vi "Append LF.vi"(0 "PDF Report IN":T21(xcontrol), 1 "Number of LF (default 1)":u8=1, 11 "error in (no error)":errorcluster) -> (4 "PDF Report duplicate":T21(xcontrol), 15 "error out":errorcluster)   [LabVIEW 2012]
doc: "Appends <B>Line Feed</B> to the PDF report.\n\n<B>FRANÇAIS</B>\nAjoute des <B>sauts de ligne</B> au rapport PDF.\n\nDeveloped by Jean-Marc Simard\nCopyright © 2010, Exaprom Inc.\nAll rights reserved.\nLicense: BSD\n\nWith iTextSharp 4.1.6 (http://itextsharp.sourceforge.net)\nunder Mozilla Public License Version 1.1\n(http://www.mozilla.org/MPL/MPL-1.1.html)"
uses:
  Controls/PDF Report Xcontrol/PDF Report.xctl
  C:/Users/MaxCorp/Documents/TopPerm - Base/DLL/itextsharp.dll
  DLL/itextsharp.dll
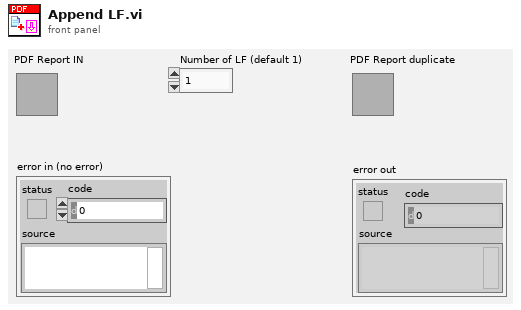
[diagram p1: front panel]
types:
  T1 = typedef "Font cluster.ctl" = cluster{"Name":string, "Size":T2, "Color":T3, "Style":cluster{"Bold":bool, "Italic":bool, "Underline":bool, "Strikeout":bool}}
  T2 = typedef "Font size.ctl" = sgl
  T3 = typedef "Font color.ctl" = u32
  T4 = typedef "Unit.ctl" = enum16{"inch", "mm"}
  T5 = typedef "Paragraphe cluster.ctl" = cluster{" Aligment":T6, "Line spacing":T7}
  T6 = typedef "Texte alignement.ctl" = enum16{"Select", "CENTER", "JUSTIFY", "LEFT", "RIGHT"}
  T7 = typedef "Line spacing.ctl" = enum16{"Select", "1.0", "1.5", "2.0"}
  T8 = typedef "Page dimensions.ctl" = cluster{"Start at page":i32, "Orientation":T9, "widht":sgl, "height":sgl, "Margin left":sgl, "Margin right":sgl, "Margin top":sgl, "Margin bottom":sgl}
  T9 = typedef "Page Orientation.ctl" = enum16{"Portrait", "Landscape"}
  T10 = typedef "Image or Table Caption.ctl" = cluster{"Caption":string, "Separator":string, "Position":enum16{"Above", "Below"}}
  T11 = typedef "Header Footer [ ].ctl" = T12[]
  T12 = typedef "Header Footer cluster.ctl" = cluster{"Start page":i32, "Type":T13, "Alignment":T14, "Vertical Alignement":T15, "Image (%)":sgl, "Page #":T16, "Text":string, "Path":string, "Font":T1, "Font refnum":refnum<k24>, "Line":cluster{"Line":T17, "Thickness (points)":sgl, "Colour":T3}}
  T13 = typedef "Header Footer Type.ctl" = enum16{"Select", "Text", "Text + hyperlink", "Page number", "Image", "Image + hyperlink"}
  T14 = typedef "Header footer horiz alignment.ctl" = enum16{"Left", "Center", "Right"}
  T15 = typedef "Cell Vertical alignment.ctl" = enum16{"TOP", "MIDDLE", "BOTTOM"}
  T16 = typedef "Page number.ctl" = cluster{"Text 1":string, "Text 2":string, "Text 3":string}
  T17 = typedef "Header Footer Line.ctl" = enum16{"No line", "Horizontal line"}
  T18 = typedef "Watermark cluster2.ctl" = cluster{"Show? (F)":bool, "Type":enum16{"Image", "Text"}, "Opacity (%)":sgl, "Rotate(°)":sgl, "Position":cluster{"Position":T19, "X":sgl, "Y":sgl}, "Image path":path, "Scaled(%)":sgl, "Image refnum":refnum<k24>, "Text":string, "Font":cluster{"Name":string, "Size":T2, "Color":T3}, "Font refnum":refnum<k24>, "Alignment":T14, "Automatic":bool}
  T19 = typedef "Watermark Position.ctl" = enum16{"Absolute", "Center (page)", "Center (text section)"}
  T20 = typedef "System Fonts.ctl" = cluster{"Font name [ ]":string[], "Font and file names [ ]":cluster{"Font name":string, "File name":string}[]}
  T21 = cluster{"Document":refnum<k24>, "Writer":refnum<k24>, "Default Font":refnum<k24>, "Default Font cluster":T1, "Path":path, "Unit (default = mm)":T4, "Paragraphe cluster":T5, "Pages dimensions [ ]":T8[], "Captions":cluster{"Image":T10, "Image counter":u16, "Table":T10, "Table counter":u16, "Font":T1}, "Header":T11, "Footer":T11, "Watermark ":T18, "Actual VI name":string, "System Fonts":T20}
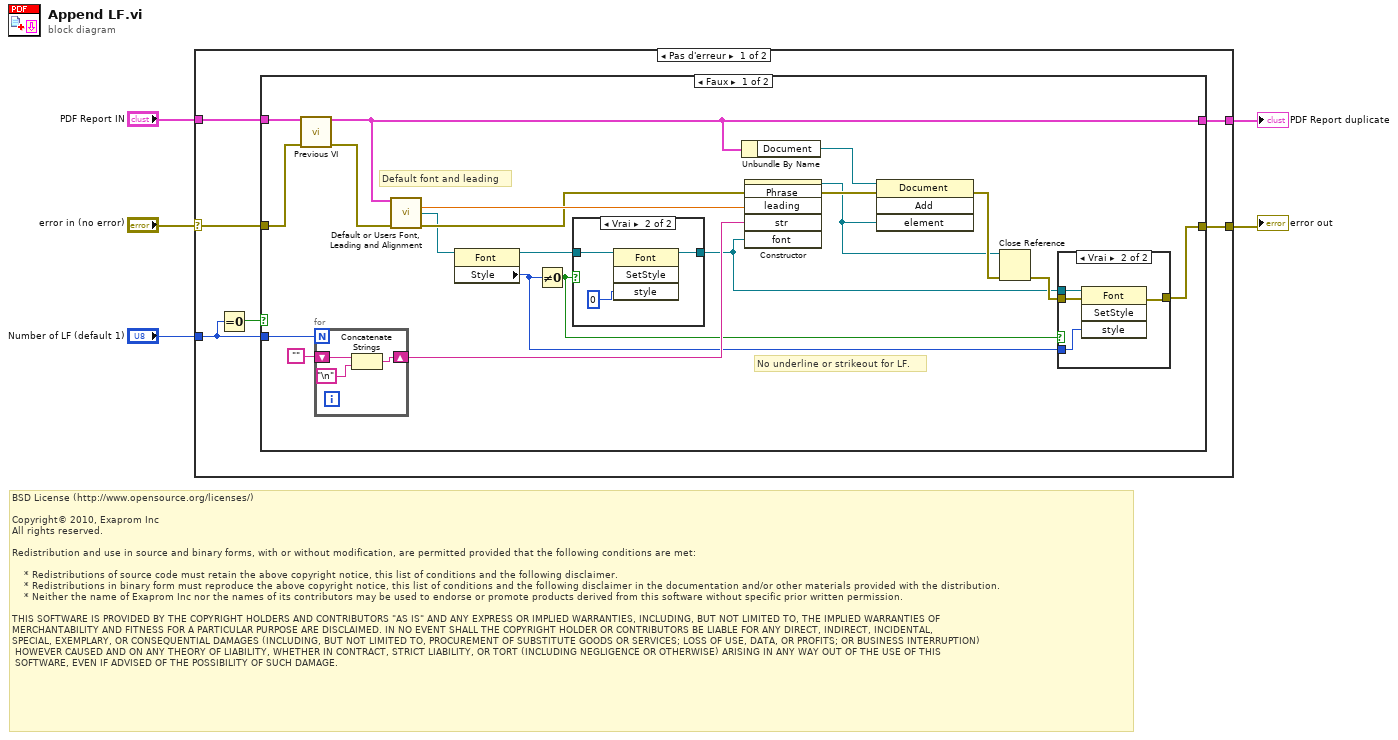
[diagram p0: block diagram]
diagram:
  # "BSD License (http://www.opensource.org/licenses/)\n\nCopyright© 2010, Exaprom Inc\nAll rights reserved.\n\nRedistribution and use in source and binary forms, with or without modification, are permitted provided that the following conditions are met:\n\n    * Redistributions of source code must retain the above copyright notice, this list of conditions and the following disclaimer.\n    * Redistributions in binary form must reproduce the above copyright notice, this list of conditions and the following disclaimer in the documentation and/or other materials provided with the distribution.\n    * Neither the name of Exaprom Inc nor the names of its contributors may be used to endorse or promote products derived from this software without specific prior written permission.\n\nTHIS SOFTWARE IS PROVIDED BY THE COPYRIGHT HOLDERS AND CONTRIBUTORS \"AS IS\" AND ANY EXPRESS OR IMPLIED WARRANTIES, INCLUDING, BUT NOT LIMITED TO, THE IMPLIED WARRANTIES OF \nMERCHANTABILITY AND FITNESS FOR A PARTICULAR PURPOSE ARE DISCLAIMED. IN NO EVENT SHALL THE COPYRIGHT HOLDER OR CONTRIBUTORS BE LIABLE FOR ANY DIRECT, INDIRECT, INCIDENTAL,\nSPECIAL, EXEMPLARY, OR CONSEQUENTIAL DAMAGES (INCLUDING, BUT NOT LIMITED TO, PROCUREMENT OF SUBSTITUTE GOODS OR SERVICES; LOSS OF USE, DATA, OR PROFITS; OR BUSINESS INTERRUPTION)\n HOWEVER CAUSED AND ON ANY THEORY OF LIABILITY, WHETHER IN CONTRACT, STRICT LIABILITY, OR TORT (INCLUDING NEGLIGENCE OR OTHERWISE) ARISING IN ANY WAY OUT OF THE USE OF THIS\n SOFTWARE, EVEN IF ADVISED OF THE POSSIBILITY OF SUCH DAMAGE."
  n1 = case shown="Pas d'erreur" "error in (no error)" {
    selector: "error in (no error)" -> [w10 w47]
    tunnel: [w11 w46] -> w2
    tunnel: [w8 w47] -> w5
    tunnel: "PDF Report IN" -> [w9 w46]
    tunnel: "Number of LF (default 1)" -> [w7 _]
    frame No Error {
      n2 = Equal To 0?(x=w7) -> (x = 0?=w6:bool)
      n3 = case shown="Faux" w6 {
        tunnel: [w12 w45] -> w11
        tunnel: w10 -> [w31 w44]
        tunnel: w9 -> [w23 w45]
        tunnel: [w21 w44] -> w8
        tunnel: w7 -> [w17 _]
        frame False {
          # "Default font and leading"
          # "No underline or strikeout for LF."
          n4 = call "Previous VI.vi"("PDF Report IN"=w23, "error in (no error)"=w31) -> ("PDF Report OUT"=w12:T21, "error out"=w30:errorcluster)  [unwired: 12 out]
          n5 = for {
            N: w17 -> [_]
            shift-right: [w38] -> w16
            shift-left: "" -> [w37]
            n6 = Concatenate Strings(w37, "\n") -> (w38:string)
          }
          n7 = call "Default or Users Font, Leading and Alignment.vi"("PDF Report"=w12, "error in (no error)"=w30) -> ("Leading"=w27:T2, "Font Ref"=w20:refnum<k24>, "error out"=w26:errorcluster)  [unwired: 2 in, 9 out]
          n8 = property class="Font"(reference=w20) -> (reference out=w19:refnum<k24>, "Style"=w14:i32)  [unwired: 1 in, 1 out]
          n9 = Not Equal To 0?(x=w14) -> (x != 0?=w13:bool)
          n10 = case shown="Vrai" w13 {
            tunnel: w19 -> [w32 w34]
            tunnel: [w32 w33] -> w15
            frame False {
            }
            frame True {
              n11 = invoke class="Font" method="SetStyle"(reference=w34, "style"=0) -> (reference out=w33:refnum<k24>)  [unwired: 2 in, 3 out]
            }
          }
          n12 = Unbundle By Name(w12) -> ("Document"=w28:refnum<k24>)
          n13 = constructor class="Phrase"(error in=w26, "leading"=w27, "str"=w16, "font"=w15) -> (reference out=w24:refnum<k24>, error out=w25:errorcluster)  [unwired: 2 in, 4 out]
          n14 = invoke class="Document" method="Add"(reference=w28, error in=w25, "element"=w24) -> (error out=w29:errorcluster)  [unwired: 1 in, 3 out]
          n15 = Close Reference(reference=w24, error in (no error)=w29) -> (error out=w22:errorcluster)
          n16 = case shown="Vrai" w13 {
            tunnel: w22 -> [w39 w43]
            tunnel: [w39 w42] -> w21
            tunnel: w14 -> [_ w41]
            tunnel: w15 -> [_ w40]
            frame False {
            }
            frame True {
              n17 = invoke class="Font" method="SetStyle"(reference=w40, error in=w43, "style"=w41) -> (error out=w42:errorcluster)  [unwired: 1 in, 3 out]
            }
          }
        }
        frame True {
        }
      }
    }
    frame Error {
    }
  }
  "error out" <- w5
  "PDF Report duplicate" <- w2
